vi "DFD FXP Postprocessing.vi"   [LabVIEW 2017, in "NI_DigFilterLicensed.lvlib"]
doc: "Converts the output signal of a fixed-point filter from a fixed-point integer representation to a floating-point representation. You must manually select the polymorphic instance you want to use."
uses:
  <vilib>/addons/Digital Filter Design/NI_DigFilterLicensed.lvlib
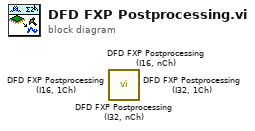
[diagram p0: block diagram]
diagram:
  n1 = call <vilib>:"DFD FXP Postprocessing (I32, nCh).vi"() -> ()  [unwired: 9 in, 3 out]
  n2 = call <vilib>:"DFD FXP Postprocessing (I16, nCh).vi"() -> ()  [unwired: 9 in, 3 out]
  n3 = call <vilib>:"DFD FXP Postprocessing (I16, 1Ch).vi"() -> ()  [unwired: 10 in, 2 out]
  n4 = call <vilib>:"DFD FXP Postprocessing (I32, 1Ch).vi"() -> ()  [unwired: 10 in, 2 out]
